vi "TxPkt - Init Packet Page.vi"(7 "Tx Packets Cluster In":T1, 8 "error in (no error)":errorcluster, 11 "Node Ptr In":T2 format="%.0x") -> (0 "error out":errorcluster, 3 "Node Ptr Out":T2 format="%.0x", 5 "Tx Packets Cluster Out":T1)   [LabVIEW 2016, in "UDP-Custom-Device System Explorer.lvlib"]
uses:
  UDP-Custom-Device System Explorer.lvlib
  <vilib>/NI Veristand/Custom Device API/Custom Device Item Ref.ctl
  Types/Page References/Refs - Tx Packets Page.ctl
  <vilib>/NI VeriStand/Custom Device API/Custom Device API.lvlib
  Property Accessors/Tx Packet Accessors.lvlib
  Property Accessors/Shared Packet Accessors.lvlib
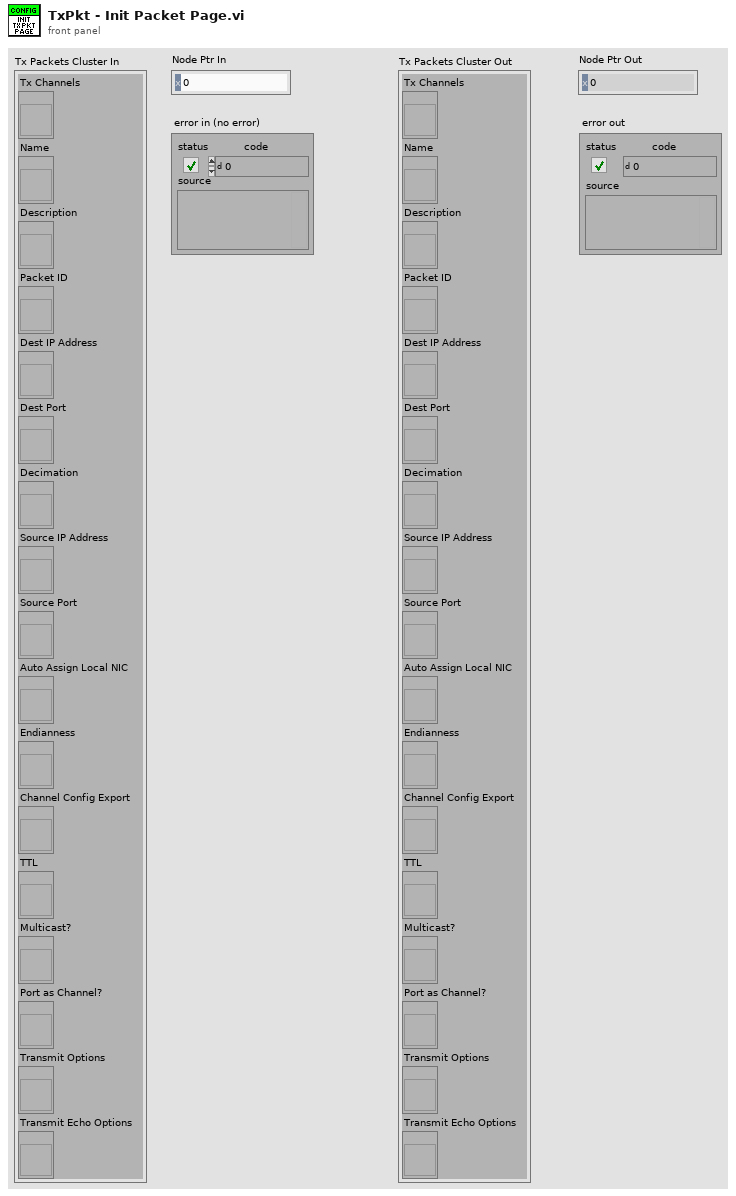
[diagram p1: front panel]
types:
  T1 = typedef "UDP-Custom-Device System Explorer.lvlib/Refs - Tx Packets Page.ctl" = cluster{"Tx Channels":refnum<vi>, "Name":refnum<vi>, "Description":refnum<vi>, "Packet ID":refnum<vi>, "Dest IP Address":refnum<vi>, "Dest Port":refnum<vi>, "Decimation":refnum<vi>, "Source IP Address":refnum<vi>, "Source Port":refnum<vi>, "Auto Assign Local NIC":refnum<vi>, "Endianness":refnum<vi>, "Channel Config Export":refnum<vi>, "TTL":refnum<vi>, "Multicast?":refnum<vi>, "Port as Channel?":refnum<vi>, "Transmit Options":refnum<vi>, "Transmit Echo Options":refnum<vi>}
  T2 = typedef "Custom Device API.lvlib/Custom Device Item Ref.ctl" = u64
  T3 = enum8{"Enabled", "Disabled", "Disabled and Grayed Out"}
  T4 = typedef "UDP-Custom-Device Shared.lvlib/Shared - Transmit Echo Options.ctl" = enum16{"PCL Reset", "Counter", "Mirror"}
  T5 = typedef "UDP-Custom-Device Shared.lvlib/Shared - Transmit Flag Options.ctl" = enum16{"Always", "One-Shot", "Toggle"}
  T6 = typedef "Custom Device API.lvlib/Custom Device Item Info.ctl" = cluster{"Name":string, "Is Channel":bool, "GUID":string, "Is Waveform":bool}
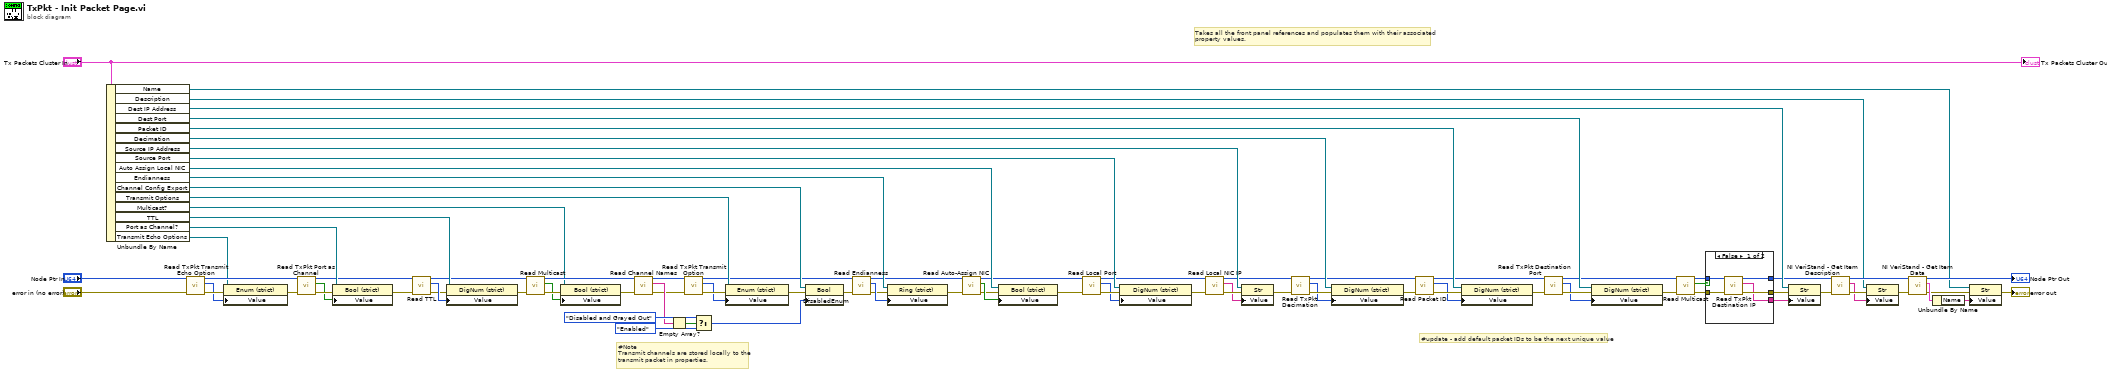
[diagram p0: block diagram]
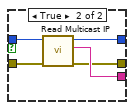
[diagram p2: hidden frame]
diagram:
  # "#Note\nTransmit channels are stored locally to the\ntransmit packet in properties."
  # "Takes all the front panel references and populates them with their associated\nproperty values."
  # "#update - add default packet IDs to be the next unique value"
  n1 = Unbundle By Name("Tx Packets Cluster In") -> ("Name"=w77:refnum<vi>, "Description"=w78:refnum<vi>, "Dest IP Address"=w80:refnum<vi>, "Dest Port"=w81:refnum<vi>, "Packet ID"=w82:refnum<vi>, "Decimation"=w76:refnum<vi>, "Source IP Address"=w75:refnum<vi>, "Source Port"=w74:refnum<vi>, "Auto Assign Local NIC"=w73:refnum<vi>, "Endianness"=w46:refnum<vi>, "Channel Config Export"=w41:refnum<vi>, "Transmit Options"=w34:refnum<vi>, "Multicast?"=w26:refnum<vi>, "TTL"=w32:refnum<vi>, "Port as Channel?"=w16:refnum<vi>, "Transmit Echo Options"=w4:refnum<vi>)
  n2 = call "Read TxPkt Transmit Echo Option.vi"("error in (no error)"="error in (no error)", "Node Ptr"="Node Ptr In") -> ("error out"=w3:errorcluster, "Transmit Echo Options"=w1:T4, "Node Ptr out"=w5:T2)  [unwired: 7 in]
  n3 = property class="Enum (strict)"(reference=w4, error in=w3, "Value"=w1) -> (error out=w2:errorcluster)  [unwired: 1 out]
  n4 = call "Read TxPkt Port as Channel.vi"("error in (no error)"=w2, "Node Ptr"=w5) -> ("error out"=w14:errorcluster, "Port as Channel"=w13:bool, "Node Ptr out"=w15:T2)  [unwired: 7 in]
  n5 = property class="Bool (strict)"(reference=w16, error in=w14, "Value"=w13) -> (error out=w17:errorcluster)  [unwired: 1 out]
  n6 = call "Read TTL.vi"("error in (no error)"=w17, "Node Ptr"=w15) -> ("error out"=w30:errorcluster, "TTL"=w31:u16, "Node Ptr out"=w29:T2)  [unwired: 7 in]
  n7 = property class="DigNum (strict)"(reference=w32, error in=w30, "Value"=w31) -> (error out=w27:errorcluster)  [unwired: 1 out]
  n8 = call "Read Multicast.vi"("error in (no error)"=w27, "Node Ptr"=w29) -> ("error out"=w25:errorcluster, "Multicast"=w23:bool, "Node Ptr out"=w28:T2)  [unwired: 7 in]
  n9 = property class="Bool (strict)"(reference=w26, error in=w25, "Value"=w23) -> (error out=w24:errorcluster)  [unwired: 1 out]
  n10 = call "Read Channel Names.vi"("error in (no error)"=w24, "Node Ptr"=w28) -> ("error out"=w9:errorcluster, "Channel Names"=w36:string[], "Node Ptr out"=w12:T2)  [unwired: 7 in]
  n11 = Empty Array?(array=w36) -> (empty?=w37:bool)
  n12 = call "Read TxPkt Transmit Option.vi"("error in (no error)"=w9, "Node Ptr"=w12) -> ("error out"=w10:errorcluster, "Transmit Options"=w8:T5, "Node Ptr out"=w11:T2)  [unwired: 7 in]
  n13 = Select(t=T3."Disabled and Grayed Out" ("Disabled"), s=w37, f=T3."Enabled" ("Disabled")) -> (s? t:f=w35:T3)
  n14 = property class="Enum (strict)"(reference=w34, error in=w10, "Value"=w8) -> (error out=w33:errorcluster)  [unwired: 1 out]
  n15 = property class="Bool"(reference=w41, error in=w33, "DisabledEnum"=w35) -> (error out=w40:errorcluster)  [unwired: 1 out]
  n16 = call "Read Endianness.vi"("error in (no error)"=w40, "Node Ptr"=w11) -> ("error out"=w43:errorcluster, "Endianness"=w45:u16, "Node Ptr out"=w44:T2)  [unwired: 7 in]
  n17 = property class="Ring (strict)"(reference=w46, error in=w43, "Value"=w45) -> (error out=w42:errorcluster)  [unwired: 1 out]
  n18 = call "Read Auto-Assign NIC.vi"("error in (no error)"=w42, "Node Ptr"=w44) -> ("error out"=w70:errorcluster, "Auto-Assign NIC"=w71:bool, "Node Ptr out"=w69:T2)  [unwired: 7 in]
  n19 = property class="Bool (strict)"(reference=w73, error in=w70, "Value"=w71) -> (error out=w68:errorcluster)  [unwired: 1 out]
  n20 = call "Read Local Port.vi"("error in (no error)"=w68, "Node Ptr"=w69) -> ("error out"=w67:errorcluster, "Port"=w66:u16, "Node Ptr out"=w65:T2)  [unwired: 7 in]
  n21 = property class="DigNum (strict)"(reference=w74, error in=w67, "Value"=w66) -> (error out=w64:errorcluster)  [unwired: 1 out]
  n22 = call "Read Local NIC IP.vi"("error in (no error)"=w64, "Node Ptr"=w65) -> ("error out"=w63:errorcluster, "IP Address of Local NIC"=w62:string, "Node Ptr out"=w61:T2)  [unwired: 7 in]
  n23 = property class="Str"(reference=w75, error in=w63, "Value"=w62) -> (error out=w60:errorcluster)  [unwired: 1 out]
  n24 = call "Read TxPkt Decimation.vi"("error in (no error)"=w60, "Node Ptr"=w61) -> ("error out"=w59:errorcluster, "Decimation"=w58:u16, "Node Ptr out"=w57:T2)  [unwired: 7 in]
  n25 = property class="DigNum (strict)"(reference=w76, error in=w59, "Value"=w58) -> (error out=w56:errorcluster)  [unwired: 1 out]
  n26 = call "Read Packet ID.vi"("error in (no error)"=w56, "Node Ptr"=w57) -> ("error out"=w55:errorcluster, "Packet ID"=w54:i32, "Node Ptr out"=w53:T2)  [unwired: 7 in]
  n27 = property class="DigNum (strict)"(reference=w82, error in=w55, "Value"=w54) -> (error out=w52:errorcluster)  [unwired: 1 out]
  n28 = call "Read TxPkt Destination Port.vi"("error in (no error)"=w52, "Node Ptr"=w53) -> ("error out"=w51:errorcluster, "Destination Port"=w50:u16, "Node Ptr out"=w20:T2)  [unwired: 7 in]
  n29 = property class="DigNum (strict)"(reference=w81, error in=w51, "Value"=w50) -> (error out=w22:errorcluster)  [unwired: 1 out]
  n30 = call "Read Multicast.vi"("error in (no error)"=w22, "Node Ptr"=w20) -> ("error out"=w21:errorcluster, "Multicast"=w18:bool, "Node Ptr out"=w19:T2)  [unwired: 7 in]
  n31 = case shown="False" w18 {
    tunnel: [w96 w99] -> w49
    tunnel: [w95 w97] -> w48
    tunnel: [w94 w98] -> w47
    tunnel: w21 -> [w93 w100]
    tunnel: w19 -> [w92 w101]
    frame False {
      n32 = call "Read TxPkt Destination IP.vi"("error in (no error)"=w93, "Node Ptr"=w92) -> ("error out"=w95:errorcluster, "Destination IP"=w94:string, "Node Ptr out"=w96:T2)  [unwired: 7 in]
    }
    frame True {
      n33 = call "Read Multicast IP.vi"("error in (no error)"=w100, "Node Ptr"=w101) -> ("error out"=w97:errorcluster, "Multicast IP Address"=w98:string, "Node Ptr out"=w99:T2)  [unwired: 7 in]
    }
  }
  n34 = property class="Str"(reference=w80, error in=w48, "Value"=w47) -> (error out=w72:errorcluster)  [unwired: 1 out]
  n35 = call <vilib>:"NI VeriStand - Get Item Description.vi"("error in (no error)"=w72, "Item Ref in"=w49) -> ("error out"=w89:errorcluster, "Description"=w88:string, "Item Ref out"=w86:T2)  [unwired: 7 out]
  n36 = property class="Str"(reference=w78, error in=w89, "Value"=w88) -> (error out=w87:errorcluster)  [unwired: 1 out]
  n37 = call <vilib>:"NI VeriStand - Get Item Data.vi"("error in (no error)"=w87, "Item Ref in"=w86) -> ("error out"=w90:errorcluster, "Item Info"=w91:T6, "Item Ref out"=→"Node Ptr Out":T2)  [unwired: 6 in, 1 out]
  n38 = Unbundle By Name(w91) -> ("Name"=w85:string)
  n39 = property class="Str"(reference=w77, error in=w90, "Value"=w85) -> (error out=→"error out":errorcluster)  [unwired: 1 out]
  "Tx Packets Cluster Out" <- "Tx Packets Cluster In"
